vi "Force Icon Editor to Unload.vi"() -> ()   [LabVIEW 2020]
doc: "If the Icon Editor is still in memory, the Keep IE Memory.vi is aborted to release the Icon Editor from memory."
panel:
  out "name found in memory":string
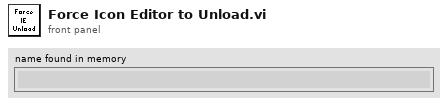
[diagram p1: front panel]
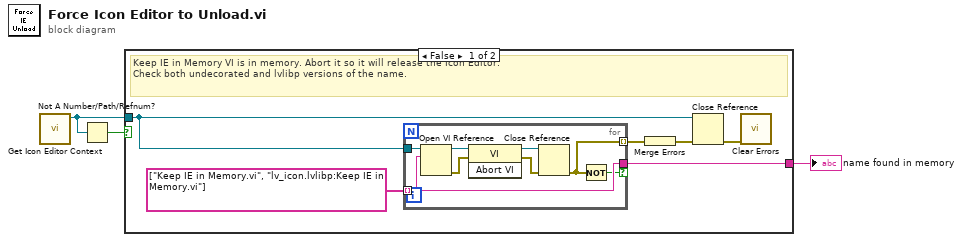
[diagram p0: block diagram]
diagram:
  n1 = call "Get Icon Editor Context.vi"() -> ("icon editor context"=w2:refnum<vi>)  [unwired: 11 in]
  n2 = Not A Number/Path/Refnum?(number/path/refnum=w2) -> (NaN/Path/Refnum?=w1:bool)
  n3 = case shown="False" w1 {
    tunnel: w2 -> [w4 _]
    tunnel: [w5 _] -> w3
    frame False {
      # "Keep IE in Memory VI is in memory. Abort it so it will release the Icon Editor.\nCheck both undecorated and lvlibp versions of the name."
      n4 = for {
        tunnel: w4 -> [w13]
        tunnel: string[] ["Keep IE in Memory.vi", "lv_icon.lvlibp:Keep IE in Memory.vi"] -> [w11] mode=indexing
        tunnel: [w15] -> w7 mode=indexing
        tunnel: [w11] -> w5 if=w10
        n5 = Open VI Reference(application reference (local)=w13, vi path=w11) -> (vi reference=w14:refnum<vi>, error out=w16:errorcluster)  [unwired: 1 in, 3 out]
        n6 = invoke class="VI" method="Abort VI"(reference=w14, error in=w16) -> (reference out=w12:refnum<vi>, error out=w17:errorcluster)  [unwired: 1 in, 1 out]
        n7 = Close Reference(reference=w12, error in (no error)=w17) -> (error out=w15:errorcluster)
        n8 = Not(x=w15) -> (.not. x?=w10:bool)
      }
      n9 = Merge Errors(w7) -> (w8:errorcluster)
      n10 = Close Reference(reference=w4, error in (no error)=w8) -> (error out=w9:errorcluster)
      n11 = call <vilib>:"Clear Errors.vi"("error in (no error)"=w9) -> ()  [unwired: 5 in, 2 out]
    }
    frame True {
    }
  }
  "name found in memory" <- w3
